vi "Main - Database (SubVI).vi"(7 "Enum":T1=enum."Write", 8 "error in (no error)":errorcluster, 11 "SQL query":string) -> (0 "error out":errorcluster, 3 "data":string[][](array[string]))   [LabVIEW 2019]
uses:
  Controls/FGV States.ctl
  <vilib>/addons/database/Connection.llb/DB Tools Open Connec (String).vi
  <vilib>/addons/database/Connection.llb/Conn Execute.vi
  <vilib>/addons/database/Recordset.llb/Rec Fetch Recordset Data (R).vi
  <vilib>/addons/database/Recordset.llb/Rec Destroy - Connection.vi
  <vilib>/addons/database/NI_Database_API.lvlib
panel:
  # "INSERT INTO `machine`(`name`, `displacement`, `transducer`, `motor`, `maxload`) VALUES ('abc','motor1','td1','motor1','12.111')"
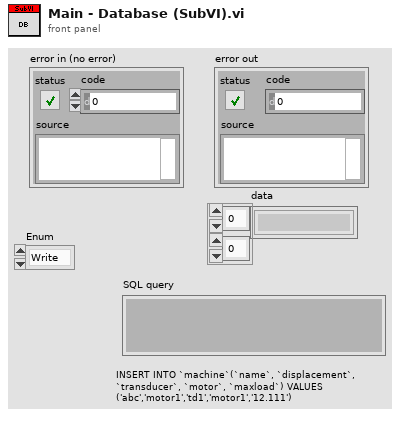
[diagram p1: front panel]
types:
  T1 = typedef "FGV States.ctl" = enum16{"Read", "Write"}
  T2 = typedef "NI_Database_API.lvlib/Conn ObjectReference.ctl" = refnum<k1>
  T3 = typedef "NI_Database_API.lvlib/Rec ObjectReference.ctl" = refnum<k1>
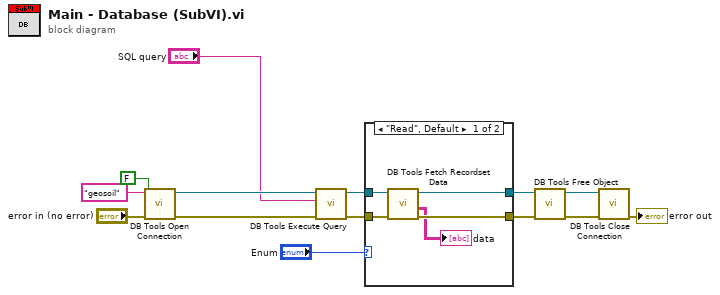
[diagram p0: block diagram]
diagram:
  n1 = call-poly <vilib>:"DB Tools Open Connection.vi"("error in (no error)"="error in (no error)", "prompt? (F)"=FALSE, "connection information"="geosoil") -> ("error out"=w8:errorcluster, "connection reference"=w12:T2)  [unwired: 5 in]
  n2 = call-poly <vilib>:"DB Tools Execute Query.vi"("error in (no error)"=w8, "SQL query"="SQL query", "connection reference"=w12) -> ("error out"=w6:errorcluster, "recordset reference"=w5:T3)  [unwired: 5 in]
  n3 = case shown="\"Read\", Default" "Enum" {
    tunnel: w6 -> [w19 w20]
    tunnel: [w18 w20] -> w2
    tunnel: w5 -> [w17 w21]
    tunnel: [w16 w21] -> w4
    frame "Read", Default {
      n4 = call-poly <vilib>:"DB Tools Fetch Recordset Data.vi"("error in (no error)"=w19, "recordset reference"=w17) -> ("error out"=w18:errorcluster, "recordset data"=→"data":string[][], "recordset reference out"=w16:T3)  [unwired: 2 in, 1 out]
    }
    frame "Write" {
    }
  }
  n5 = call-poly <vilib>:"DB Tools Free Object.vi"("error in (no error)"=w2, "recordset reference"=w4) -> ("error out"=w9:errorcluster, "connection reference"=w13:T2)  [unwired: 8 in]
  n6 = call <vilib>:"DB Tools Close Connection.vi"("error in (no error)"=w9, "connection reference"=w13) -> ("error out"=→"error out":errorcluster)  [unwired: 5 in]
